vi "计算散斑矩阵列平均值.vi"(1 "光源散斑簇":T1) -> (0 "散斑二维数组列平均值":dbl[](array[numeric]))   [LabVIEW 2018]
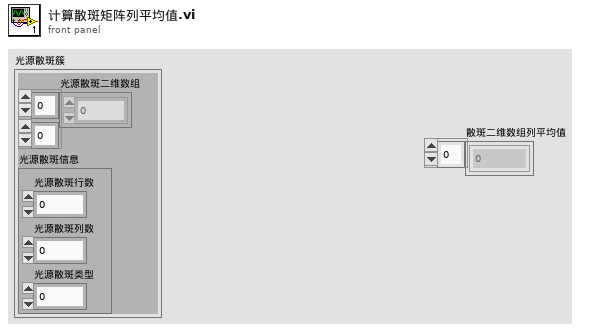
[diagram p1: front panel]
types:
  T1 = cluster{"光源散斑二维数组":dbl[][], "光源散斑信息":cluster{"光源散斑行数":dbl, "光源散斑列数":dbl, "光源散斑类型":dbl}}
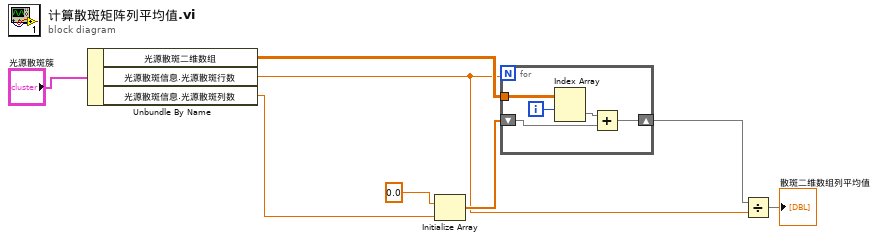
[diagram p0: block diagram]
diagram:
  n1 = Unbundle By Name("光源散斑簇") -> ("光源散斑二维数组"=w4:dbl[][], "光源散斑信息.光源散斑行数"=w3:dbl, "光源散斑信息.光源散斑列数"=w2:dbl)
  n2 = Initialize Array(0.0, w2) -> (w6:dbl[])
  n3 = for {
    N: w3 -> [_]
    shift-right: [w9] -> w8
    shift-left: w6 -> [w10]
    tunnel: w4 -> [w13]
    i -> [w12]
    n4 = Index Array(array=w13, index (row)=w12) -> (element=w11:dbl[])  [unwired: 1 in]
    n5 = Add(x=w11, y=w10) -> (x+y=w9:dbl[])
  }
  n6 = Divide(x=w8, y=w3) -> (x/y=→"散斑二维数组列平均值":dbl[])
